vi "Get Number of Steps.vi"(8 "error in (no error)":errorcluster, 11 "Ramp Use Case in":refnum<class "Ramp Voltage.lvclass">) -> (0 "error out":errorcluster, 2 "Numeric":i32, 3 "Ramp Use Case out":refnum<class "Ramp Voltage.lvclass">)   [LabVIEW 2020, in "High Level PSU With Tests.lvlib" / "Ramp Voltage.lvclass"]
uses:
  Ramp Voltage.lvclass
  Ramp Voltage.lvclass/Ramp Voltage.ctl
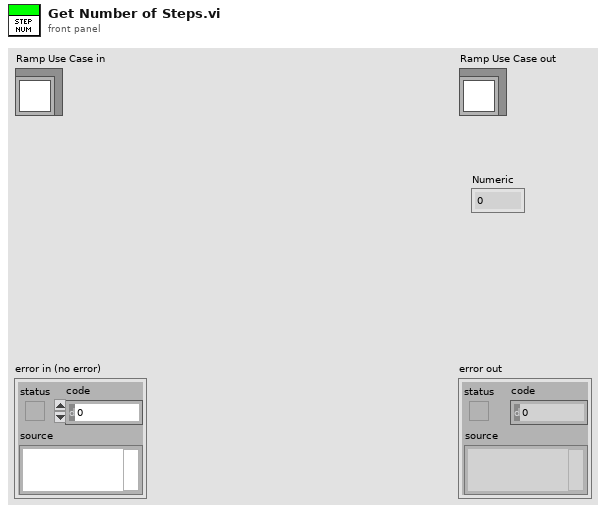
[diagram p1: front panel]
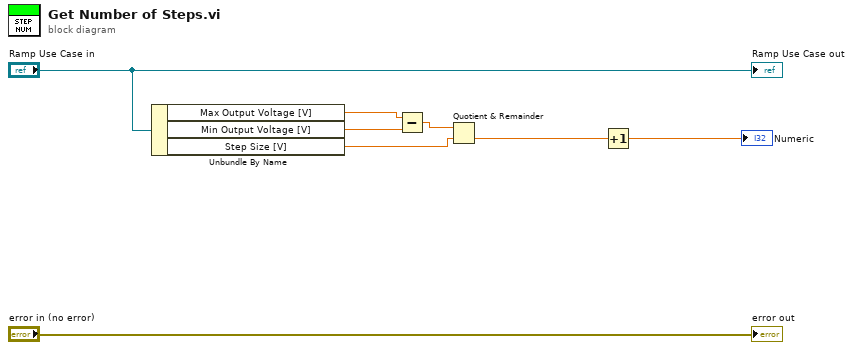
[diagram p0: block diagram]
diagram:
  n1 = Unbundle By Name("Ramp Use Case in") -> ("Max Output Voltage [V]"=w6:dbl, "Min Output Voltage [V]"=w5:dbl, "Step Size [V]"=w3:dbl)
  n2 = Subtract(x=w6, y=w5) -> (x-y=w4:dbl)
  n3 = Quotient & Remainder(x=w4, y=w3) -> (floor(x/y)=w2:dbl)  [unwired: 1 out]
  n4 = Increment(x=w2) -> (x+1=→"Numeric":dbl)
  "error out" <- "error in (no error)"
  "Ramp Use Case out" <- "Ramp Use Case in"
